vi "ROIsToPoints.vi"(9 "GridPoints":dbl=5.0, 10 "Scan Settings":T2, 11 "ROI":T1(array[cluster])) -> (1 "Number of motion points":i32, 2 "Number of points":i32, 3 "Points":i32[][](array[numeric]))   [LabVIEW 2012]
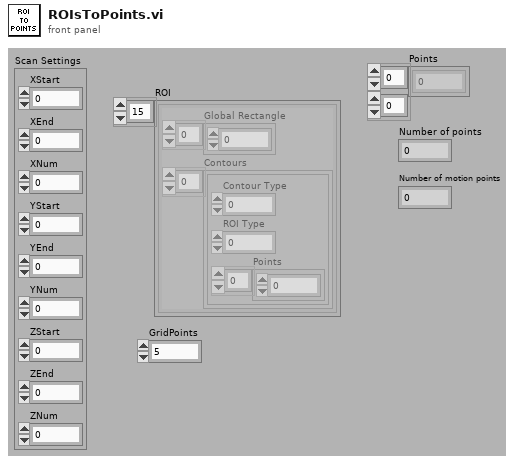
[diagram p1: front panel]
types:
  T1 = cluster{"Global Rectangle":i32[], "Contours":cluster{"Contour Type":u32, "ROI Type":u32, "Points":i32[]}[]}[]
  T2 = cluster{"XStart":i32, "XEnd":i32, "XNum":i32, "YStart":i32, "YEnd":i32, "YNum":i32, "ZStart":i32, "ZEnd":i32, "ZNum":i32}
  T3 = cluster{"Contour Type":u32, "ROI Type":u32, "Points":i32[]}[]
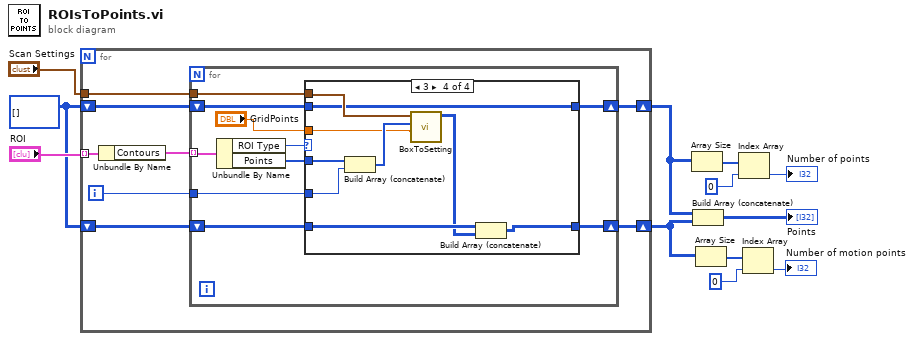
[diagram p0: block diagram]
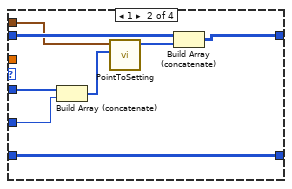
[diagram p3: hidden frame]
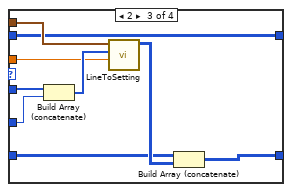
[diagram p4: hidden frame]
diagram:
  w7 = i32[][] []
  n1 = for {
    tunnel: "ROI" -> [w20] mode=indexing
    shift-right: [w16] -> w6
    shift-left: w7 -> [w17]
    tunnel: "Scan Settings" -> [w15]
    shift-right: [w13] -> w2
    shift-left: w7 -> [w14]
    i -> [w18]
    n2 = Unbundle By Name(w20) -> ("Contours"=w19:T3)
    n3 = for {
      tunnel: w19 -> [w30] mode=indexing
      tunnel: w18 -> [w26]
      shift-right: [w25] -> w16
      shift-left: w17 -> [w27]
      tunnel: w15 -> [w24]
      shift-right: [w21] -> w13
      shift-left: w14 -> [w22]
      n4 = Unbundle By Name(w30) -> ("ROI Type"=w29:u32, "Points"=w28:i32[])
      n5 = case shown="3" w29 {
        tunnel: w28 -> [_ w40 w49 w57]
        tunnel: w27 -> [w32 w38 w41 w50]
        tunnel: w26 -> [_ w39 w48 w58]
        tunnel: [w32 w37 w41 w50] -> w25
        tunnel: w24 -> [_ w35 w47 w56]
        tunnel: "GridPoints" -> [_ _ w45 w54]
        tunnel: w22 -> [w31 w33 w43 w53]
        tunnel: [w31 w33 w42 w52] -> w21
        frame 0, Default {
        }
        frame 1 {
          n6 = Build Array (concatenate)(w40, w39) -> (w34:i32[])
          n7 = call "PointToSetting.vi"("Clicked"=w34, "Scan Settings"=w35) -> ("Setting"=w36:i32[])  [unwired: 9 in]
          n8 = Build Array (concatenate)(w38, w36) -> (w37:i32[][])
        }
        frame 2 {
          n9 = Build Array (concatenate)(w49, w48) -> (w46:i32[])
          n10 = call "LineToSetting.vi"("GridSize"=w45, "Line"=w46, "Scan Settings"=w47) -> ("Settings"=w44:i32[][])  [unwired: 8 in]
          n11 = Build Array (concatenate)(w43, w44) -> (w42:i32[][])
        }
        frame 3 {
          n12 = Build Array (concatenate)(w57, w58) -> (w55:i32[])
          n13 = call "BoxToSetting.vi"("GridSize"=w54, "Line"=w55, "Scan Settings"=w56) -> ("Settings"=w51:i32[][])  [unwired: 8 in]
          n14 = Build Array (concatenate)(w53, w51) -> (w52:i32[][])
        }
      }
    }
  }
  n15 = Array Size(array=w6) -> (size(s)=w10:i32[])
  n16 = Build Array (concatenate)(w6, w2) -> (→"Points":i32[][])
  n17 = Array Size(array=w2) -> (size(s)=w4:i32[])
  n18 = Index Array(array=w10, index=0) -> (element=→"Number of points":i32)
  n19 = Index Array(array=w4, index=0) -> (element=→"Number of motion points":i32)
